vi "get channels by classification.vi"(6 "channel classification":T2, 8 "error in":errorcluster, 11 "shared memory runtime in":refnum<class "Shared Memory Runtime.lvclass">) -> (0 "error out":errorcluster, 2 "channels":T1[](array[typedef]), 3 "shared memory runtime out":refnum<class "Shared Memory Runtime.lvclass">)   [LabVIEW 2013, in "Shared Memory Runtime.lvclass"]
uses:
  Shared Memory Runtime.lvclass
  <vilib>/NI/Tag Bus Module Framework/channel/channel classification.ctl
  shared memory module runtime.ctl
  <vilib>/NI/Tag Bus/tag/Data Type.ctl
  <vilib>/National Instruments/Shared Memory Library for Linux RT/Controls/Shared Memory Class Reference.ctl
  <vilib>/National Instruments/Shared Memory Library for Linux RT/Classes/Shared Memory/Shared Memory.lvclass
  Shared Memory Runtime.lvclass/Shared Memory Runtime.ctl
  Read input data.vi
  Read processing parameters.vi
  Read processing results.vi
  Read output data.vi
  <vilib>/NI/Tag Bus Module Framework/channel/TBM channel.lvclass
  <vilib>/NI/Tag Bus/tag/tag descriptor.lvclass
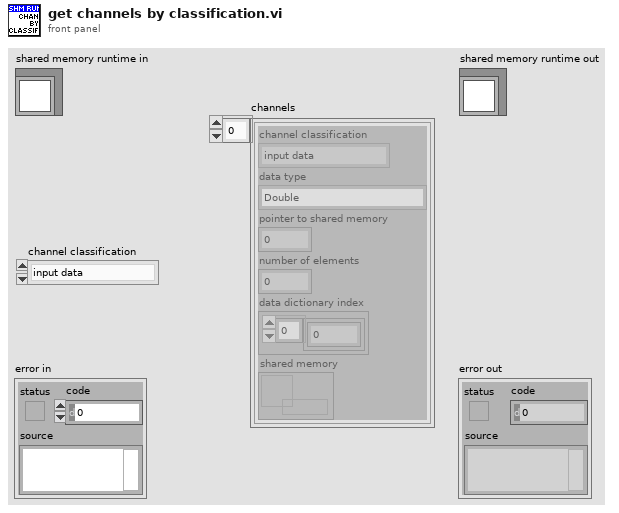
[diagram p1: front panel]
types:
  T1 = typedef "shared memory runtime.lvclass/shared memory module runtime.ctl" = cluster{"channel classification":T2, "data type":T3, "pointer to shared memory":u64, "number of elements":u64, "data dictionary index":cluster{i32[]}, "shared memory":T4}
  T2 = typedef "TBM channel.lvclass/channel classification.ctl" = enum16{"input data", "output data", "processing parameter", "processing result"}
  T3 = typedef "tag bus.lvlib/tag descriptor.lvclass/Data Type.ctl" = enum16{"Double", "Single", "I64", "I32", "I16", "I8", "U64", "U32", "U16", "U8", "Boolean", "String", "Array of Double", "Array of Single", "Array of I64", "Array of I32", "Array of I16", "Array of I8", "Array of U64", "Array of U32", "Array of U16", "Array of U8", "Array of Boolean", "Array of String"}
  T4 = typedef "Shared Memory Class Reference.ctl" = refnum<data-value>
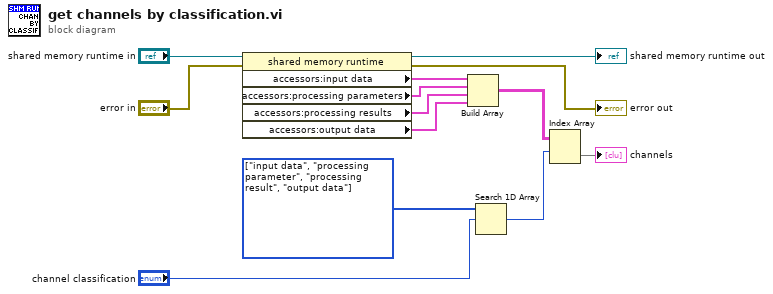
[diagram p0: block diagram]
diagram:
  w6 = T2[] [enum."input data", enum."processing parameter", enum."processing result", enum."output data"] items=["input data", "output data", "processing parameter", "processing result"] ("supported classifications")
  n1 = property class="shared memory runtime"(reference="shared memory runtime in", error in="error in") -> (reference out=→"shared memory runtime out":refnum<class "Shared Memory Runtime.lvclass">, error out=→"error out":errorcluster, "accessors:input data"=w2:T1[], "accessors:processing parameters"=w11:T1[], "accessors:processing results"=w12:T1[], "accessors:output data"=w13:T1[])
  n2 = Build Array(w2, w11, w12, w13) -> (w4:T1[][])
  n3 = Search 1D Array(1D array=w6, element="channel classification") -> (index of element=w3:i32)  [unwired: 1 in]
  n4 = Index Array(array=w4, index (row)=w3) -> (element=→"channels":T1[])  [unwired: 1 in]
